vi "State Queue PUSH.vi"(6 "Queue At Back? (T)":bool=TRUE, 7 "State case":string, 8 "error in (no error)":errorcluster, 9 "Parameters":variant, 11 "State que in":T1[](array[typedef])) -> (0 "error out":errorcluster, 3 "State que out":T1[](array[typedef]))   [LabVIEW 2013, in "State Machine Lib.lvlib"]
doc: "Pushes a states and a parameter list (array of variants) onto the state queue. Can be pushed onto the front of the queue for priority."
uses:
  State Machine Lib.lvlib
  STATE cluster.ctl
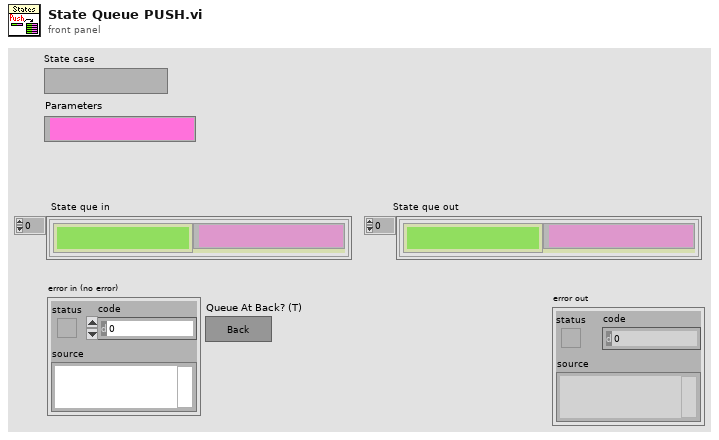
[diagram p1: front panel]
types:
  T1 = typedef "State Machine Lib.lvlib/STATE cluster.ctl" = cluster{"State":string, "Parameters":variant}
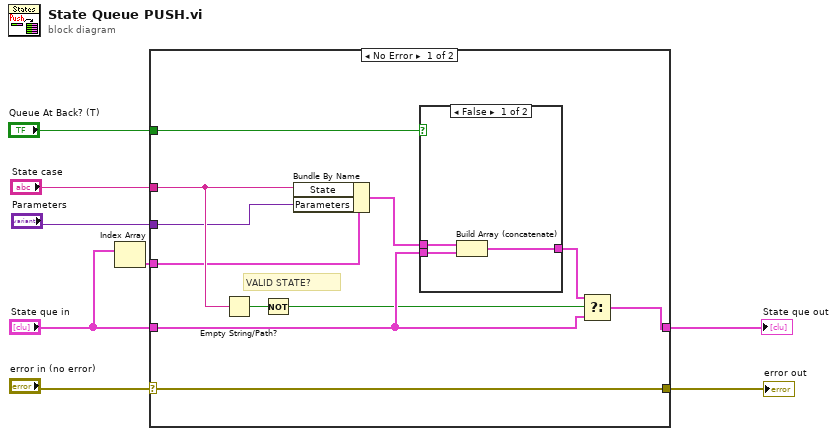
[diagram p0: block diagram]
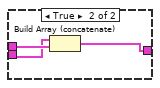
[diagram p2: hidden frame]
diagram:
  n1 = Index Array(array="State que in") -> (element=w3:T1)  [unwired: 1 in]
  n2 = case shown="No Error" "error in (no error)" {
    selector: "error in (no error)" -> [w19 w26]
    tunnel: [w19 w26] -> w7
    tunnel: [w16 w27] -> w8
    tunnel: "State que in" -> [w14 w27]
    tunnel: "Parameters" -> [w17 _]
    tunnel: "State case" -> [w18 _]
    tunnel: w3 -> [w11 _]
    tunnel: "Queue At Back? (T)" -> [w12 _]
    frame No Error {
      # "VALID STATE?"
      n3 = Empty String/Path?(string/path=w18) -> (empty?=w10:bool)
      n4 = Not(x=w10) -> (.not. x?=w9:bool)
      n5 = Bundle By Name(cluster=w11, "State"=w18, "Parameters"=w17) -> (w13:T1)
      n6 = case shown="False" w12 {
        tunnel: [w22 w23] -> w15
        tunnel: w14 -> [w21 w24]
        tunnel: w13 -> [w20 w25]
        frame False {
          n7 = Build Array (concatenate)(w20, w21) -> (w22:T1[])
        }
        frame True {
          n8 = Build Array (concatenate)(w24, w25) -> (w23:T1[])
        }
      }
      n9 = Select(t=w15, s=w9, f=w14) -> (s? t:f=w16:T1[])
    }
    frame Error {
    }
  }
  "State que out" <- w8
  "error out" <- w7
